vi "Stop Core.vi"(10 "final error code":i32 caption="最终错误代码", 11 "VoiceControl in":refnum<class "Voice.lvclass"> caption="操作者输入") -> (3 "VoiceControl out":refnum<class "Voice.lvclass"> caption="操作者输出")   [LabVIEW 2014, in "Voice.lvlib" / "Voice.lvclass"]
doc: "(<B>文件名</B>：Actor Framework.lvlib:Actor.lvclass:Stop Core.vi)\n\n定义停止前操作者的动作。使用<B>最终错误代码</B>输入判断操作者是否在出错时关闭。\n\n默认情况下，该方法不执行任何动作。子孙类重写该方法，定义出错时的操作，例如，关闭操作者核心方法初始的进程。"
uses:
  Voice.lvclass
  Voice.lvclass/Voice.ctl
  <vilib>/ActorFramework/Actor/Actor.lvclass
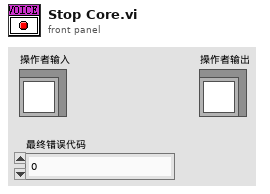
[diagram p1: front panel]
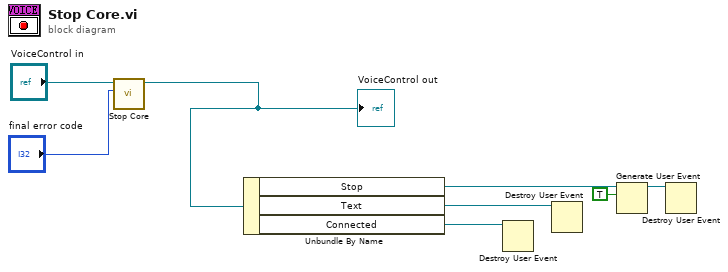
[diagram p0: block diagram]
diagram:
  n1 = call-parent "Stop Core.vi"("final error code"="final error code", "Actor in"="VoiceControl in") -> ("Actor out"=w1:refnum<class "Voice.lvclass">)  [unwired: 9 in]
  "VoiceControl out" <- w1
  n2 = Unbundle By Name(w1) -> ("Stop"=w6:refnum<user-event>, "Text"=w4:refnum<user-event>, "Connected"=w2:refnum<user-event>)
  n3 = Destroy User Event(user event=w2) -> ()  [unwired: 1 in, 1 out]
  n4 = Destroy User Event(user event=w4) -> ()  [unwired: 1 in, 1 out]
  n5 = Generate User Event(user event=w6, event data cluster=TRUE ("event data")) -> (user event out=w3:refnum<user-event>)  [unwired: 2 in, 1 out]
  n6 = Destroy User Event(user event=w3) -> ()  [unwired: 1 in, 1 out]
